vi "string.vi"(10 "in2":string, 11 "in1":string) -> (3 "output":string)   [LabVIEW 2020]
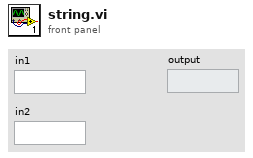
[diagram p1: front panel]
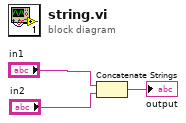
[diagram p0: block diagram]
diagram:
  n1 = Concatenate Strings("in1", "in2") -> (→"output":string)
